vi "Get Next Data.vi"(8 "error in (no error)":errorcluster, 11 "Random Data Plugin in":refnum<class "Random Data Plugin.lvclass">) -> (0 "error out":errorcluster, 2 "Data":dbl, 3 "Random Data Plugin out":refnum<class "Random Data Plugin.lvclass">)   [LabVIEW 2017, in "Data Engine.lvlib" / "Random Data Plugin.lvclass"]
uses:
  Random Data Plugin.lvclass
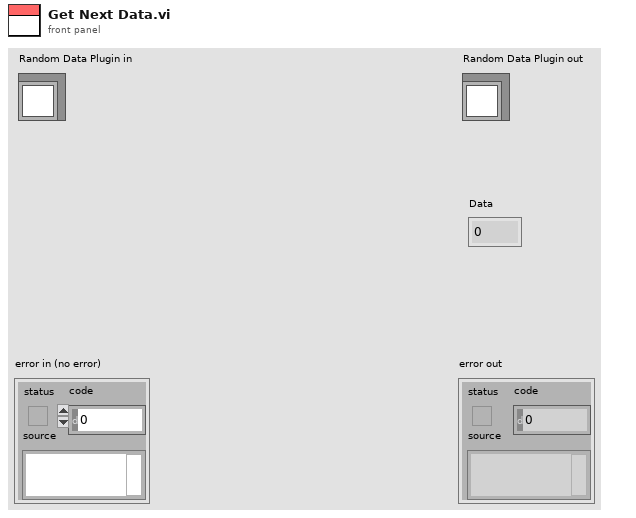
[diagram p1: front panel]
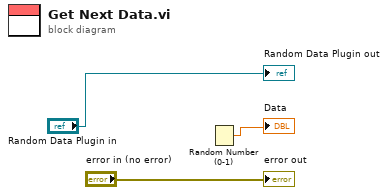
[diagram p0: block diagram]
diagram:
  n1 = Random Number (0-1)() -> (number: 0 to 1=→"Data":dbl)
  "error out" <- "error in (no error)"
  "Random Data Plugin out" <- "Random Data Plugin in"
